vi "if_v0_v4.vi"() -> ()   [LabVIEW 2009]
panel:
  out "Starea apei":string="Abur"
  in  "Temperatura":dbl(slide)=114.11960132890366 scale=-30.0..150.0
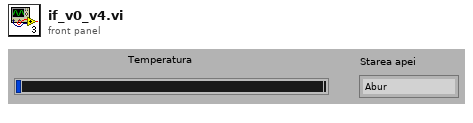
[diagram p1: front panel]
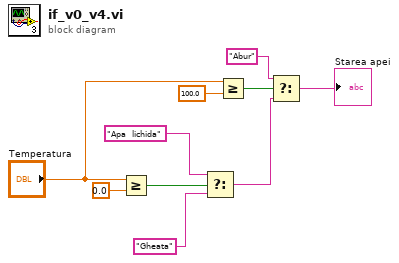
[diagram p0: block diagram]
diagram:
  n1 = Greater Or Equal?(x="Temperatura", y=0.0) -> (x >= y?=w9:bool)
  n2 = Select(t="Apa  lichida" ("Apa este lichida"), s=w9, f="Gheata") -> (s? t:f=w2:string)
  n3 = Greater Or Equal?(x="Temperatura", y=100.0) -> (x >= y?=w5:bool)
  n4 = Select(t="Abur" ("Apa este lichida"), s=w5, f=w2) -> (s? t:f=→"Starea apei":string)
